vi "Example Find Borders.vi"() -> ()   [LabVIEW 2010]
uses:
  C:/tf/play/labview/Tinkerforge.dll
panel:
  out "last border":string
  in  "stop":bool
  out "callback counter":i32
  in  "uid":string="6j9"
  in  "port":i32=4223
  in  "host":string="localhost"
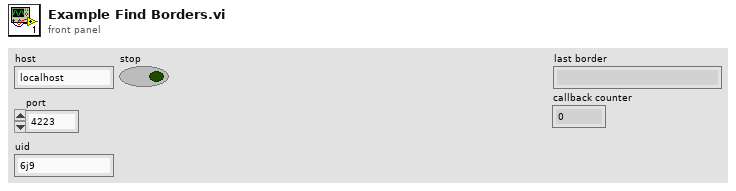
[diagram p1: front panel]
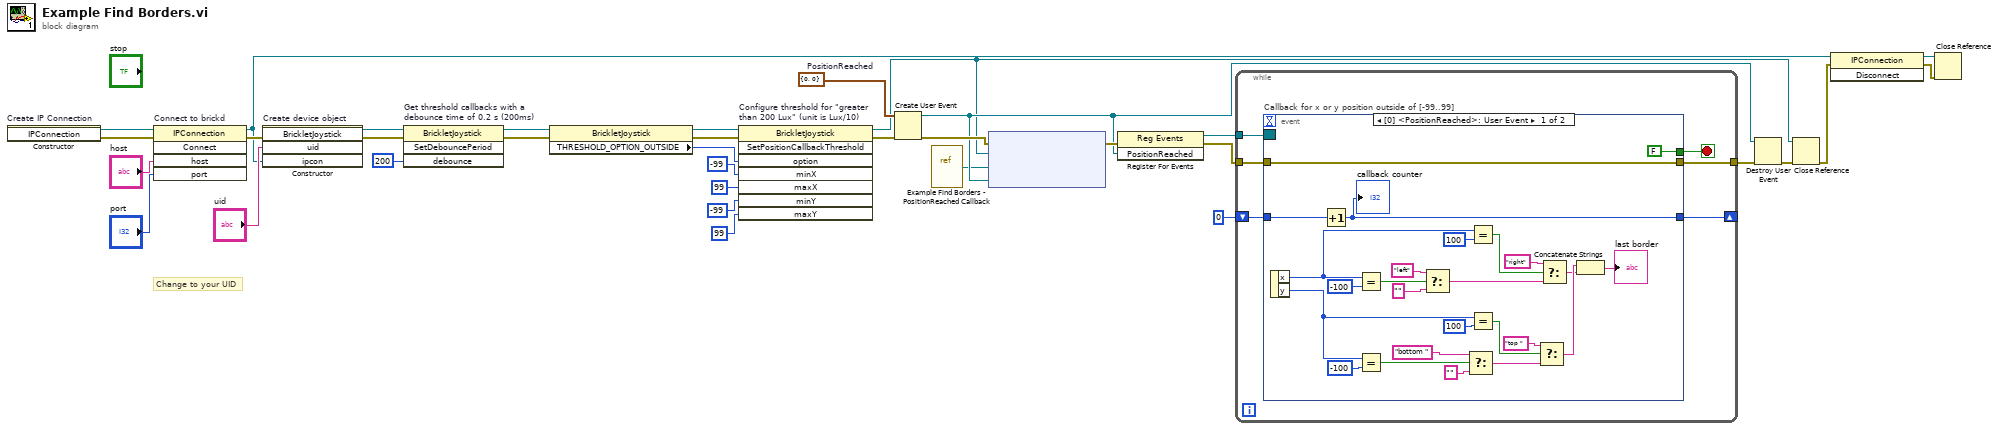
[diagram p0: block diagram]
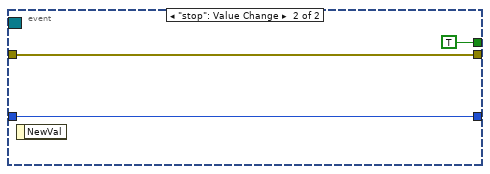
[diagram p2: hidden frame]
diagram:
  w18 = cluster{"x":i16, "y":i16} {"x"=0, "y"=0}  # PositionReached
  # "Change to your UID"
  n1 = constructor on="Create IP Connection" class="IPConnection"() -> (reference out=w34:refnum<k24>, error out=w6:errorcluster)  [unwired: 3 in, 1 out]
  n2 = invoke on="Connect to brickd" class="IPConnection" method="Connect"(reference=w34, error in=w6, "host"="host", "port"="port") -> (reference out=w27:refnum<k24>, error out=w30:errorcluster)  [unwired: 1 in, 3 out]
  n3 = constructor on="Create device object" class="BrickletJoystick"(error in=w30, "uid"="uid", "ipcon"=w27) -> (reference out=w16:refnum<k24>, error out=w17:errorcluster)  [unwired: 2 in, 3 out]
  n4 = invoke on="Get threshold callbacks with a\ndebounce time of 0.2 s (200ms)" class="BrickletJoystick" method="SetDebouncePeriod"(reference=w16, error in=w17, "debounce"=i64 200 ("period")) -> (reference out=w10:refnum<k24>, error out=w12:errorcluster)  [unwired: 1 in, 2 out]
  n5 = property class="BrickletJoystick"(reference=w10, error in=w12) -> (reference out=w9:refnum<k24>, error out=w11:errorcluster, "THRESHOLD_OPTION_OUTSIDE"=w8:u16)
  n6 = invoke on="Configure threshold for \"greater\nthan 200 Lux\" (unit is Lux/10)" class="BrickletJoystick" method="SetPositionCallbackThreshold"(reference=w9, error in=w11, "option"=w8, "minX"=i16 -99 ("min"), "maxX"=i16 99 ("max"), "minY"=i16 -99 ("min"), "maxY"=i16 99 ("max")) -> (reference out=w14:refnum<k24>, error out=w13:errorcluster)  [unwired: 1 in, 6 out]
  n7 = Create User Event(user event datatype=w18, error in=w13) -> (user event=w20:refnum<user-event>, error out=w25:errorcluster)
  n8 = vi-ref "Example Find Borders - PositionReached Callback.vi"() -> ("vi reference"=w1:refnum<vi>)
  n9 = node ("Register Event Callback")(w25, w14, w1, w20) -> (w24:errorcluster)  [unwired: 1 in, 1 out]
  n10 = register-events(error in=w24, w20) -> (reference out=w23:refnum<event-registration>, error out=w21:errorcluster)  [unwired: 1 in]
  n11 = while {
    tunnel: w23 -> [w40]
    tunnel: [w39] -> w22
    tunnel: w21 -> [w38]
    shift-right: [w36] -> _
    shift-left: 0 -> [w37]
    stop <- w35 stop-if-true
    n12 = event "Callback for x or y position outside of [-99..99]" shown="[0] <PositionReached>: User Event" {
      selector: w40 -> [_ _]
      dyn-events: _ -> [_ _]
      timeout: _ -> [_ _]
      tunnel: [w65 w67] -> w39
      tunnel: w38 -> [w65 w67]
      tunnel: w37 -> [w64 w66]
      tunnel: [w63 w66] -> w36
      tunnel: [FALSE TRUE] -> w35
      event User Event {
        n13 = event-data() -> ("x"=w42:i16, "y"=w41:i16)  [unwired: 1 in]
        n14 = Increment(x=w64) -> (x+1=w63:i32)
        "callback counter" <- w63
        n15 = Equal?(x=w42, y=i16 -100) -> (x = y?=w46:bool)
        n16 = Equal?(x=w41, y=i16 -100) -> (x = y?=w51:bool)
        n17 = Select(t="left", s=w46, f="") -> (s? t:f=w43:string)
        n18 = Select(t="bottom ", s=w51, f="") -> (s? t:f=w48:string)
        n19 = Equal?(x=w42, y=i16 100) -> (x = y?=w55:bool)
        n20 = Equal?(x=w41, y=i16 100) -> (x = y?=w60:bool)
        n21 = Select(t="top ", s=w60, f=w48) -> (s? t:f=w58:string)
        n22 = Select(t="right", s=w55, f=w43) -> (s? t:f=w53:string)
        n23 = Concatenate Strings(w58, w53) -> (→"last border":string)
      }
      event "stop": Value Change {
        n24 = event-data() -> ()  [unwired: 1 in, 1 out]
      }
    }
  }
  n25 = Destroy User Event(user event=w20, error in=w22) -> (error out=w19:errorcluster)
  n26 = Close Reference(reference=w14, error in (no error)=w19) -> (error out=w29:errorcluster)
  n27 = invoke class="IPConnection" method="Disconnect"(reference=w27, error in=w29) -> (reference out=w26:refnum<k24>, error out=w28:errorcluster)  [unwired: 1 in, 1 out]
  n28 = Close Reference(reference=w26, error in (no error)=w28) -> ()  [unwired: 1 out]
